vi "Initialize.vi"(11 "PID Loop in":refnum<class "PID Loop.lvclass">) -> (0 "error out":errorcluster, 3 "PID Loop out":refnum<class "PID Loop.lvclass">)   [LabVIEW 2024, in "PID Loop.lvlib" / "PID Loop.lvclass"]
uses:
  PID Loop.lvclass
  PID Loop.lvclass/PID Loop.ctl
  src/Zero Timeout Message Handler/Zero Timeout Message Handler/Zero Timeout Message Handler.lvclass
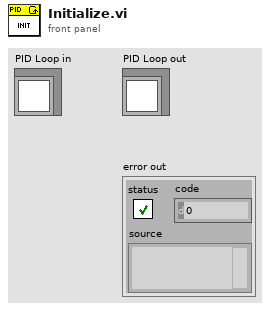
[diagram p1: front panel]
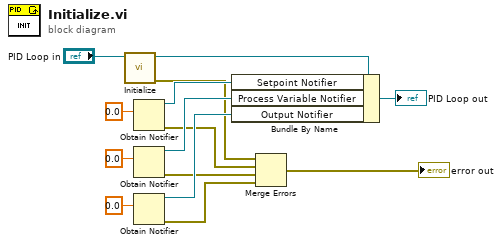
[diagram p0: block diagram]
diagram:
  n1 = call-parent "Initialize.vi"("Zero Timeout Message Handler in"="PID Loop in") -> ("error out"=w1:errorcluster, "Zero Timeout Message Handler out"=w13:refnum<class "PID Loop.lvclass">)  [unwired: 9 in]
  n2 = Obtain Notifier(notification data type=0.0) -> (notifier out=w8:refnum<notifier>, error out=w5:errorcluster)  [unwired: 3 in, 1 out]
  n3 = Obtain Notifier(notification data type=0.0) -> (notifier out=w7:refnum<notifier>, error out=w4:errorcluster)  [unwired: 3 in, 1 out]
  n4 = Obtain Notifier(notification data type=0.0) -> (notifier out=w6:refnum<notifier>, error out=w3:errorcluster)  [unwired: 3 in, 1 out]
  n5 = Bundle By Name(cluster=w13, "Setpoint Notifier"=w8, "Process Variable Notifier"=w7, "Output Notifier"=w6) -> (→"PID Loop out":refnum<class "PID Loop.lvclass">)
  n6 = Merge Errors(w1, w5, w4, w3) -> (→"error out":errorcluster)
